vi "PneumaticsMain.vi"(7 "Mode":enum16{"Open", "Control"}(ring)=enum."Control", 8 "error in (no error)":errorcluster, 9 "Value":T1, 10 "Reverse Solenoid Channel":T2=enum."Solenoid 1", 11 "Forward Solenoid Channel":T2) -> (0 "error out":errorcluster)   [LabVIEW 2017]
uses:
  <vilib>/Rock Robotics/WPI/Solenoid/WPI_SolenoidChannel.ctl
  <vilib>/Rock Robotics/WPI/Solenoid/WPI_SolenoidValue.ctl
  <vilib>/Rock Robotics/WPI/Solenoid/WPI_SolenoidOpenDouble.vi
  <vilib>/Rock Robotics/WPI/Solenoid/WPI_SolenoidSetEnum.vi
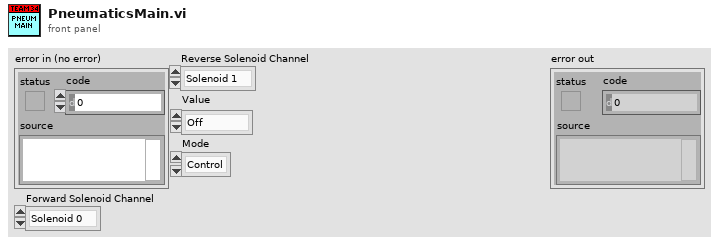
[diagram p1: front panel]
types:
  T1 = typedef "WPI_SolenoidValue.ctl" = enum16{"Off", "On", "Forward", "Reverse"}
  T2 = typedef "WPI_SolenoidChannel.ctl" = enum8{"Solenoid 0", "Solenoid 1", "Solenoid 2", "Solenoid 3", "Solenoid 4", "Solenoid 5", "Solenoid 6", "Solenoid 7", "Invalid"}
  T3 = typedef "WPI_SolenoidDevRef.ctl" = cluster{"DevStatus":errorcluster, "Pneumatics Control Module":u8, "Forward Solenoid Channel":T2, "Reverse Solenoid Channel":T2}
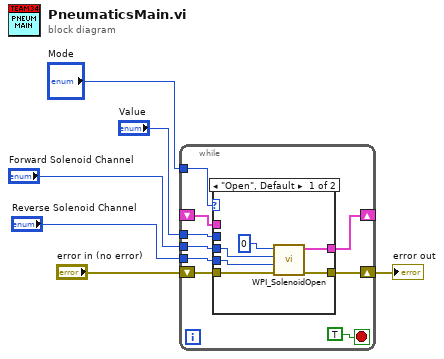
[diagram p0: block diagram]
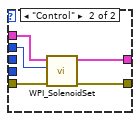
[diagram p2: hidden frame]
diagram:
  n1 = while {
    tunnel: "Mode" -> [w15]
    tunnel: "Forward Solenoid Channel" -> [w13]
    tunnel: "Reverse Solenoid Channel" -> [w12]
    shift-right: [w11] -> _
    shift-left: _ -> [w9]
    tunnel: "Value" -> [w10]
    shift-right: [w14] -> w5
    shift-left: "error in (no error)" -> [w8]
    stop <- TRUE stop-if-true
    n2 = case shown="\"Open\", Default" w15 {
      tunnel: [w20 w23] -> w14
      tunnel: w13 -> [w19 _]
      tunnel: w12 -> [w18 _]
      tunnel: [w17 w24] -> w11
      tunnel: w10 -> [_ w26]
      tunnel: w9 -> [_ w25]
      tunnel: w8 -> [w16 w22]
      frame "Open", Default {
        n3 = call-poly <vilib>:"WPI_SolenoidOpen.vi"("error in (no error)"=w16, "Reverse Solenoid Channel"=w18, "Forward Solenoid Channel"=w19, "Pneumatics Control Module (0)"=u8 0) -> ("error out"=w20:errorcluster, "SolenoidDevRef"=w17:T3)  [unwired: 6 in]
      }
      frame "Control" {
        n4 = call-poly <vilib>:"WPI_SolenoidSet.vi"("error in (no error)"=w22, "Value"=w26, "SolenoidDevRef"=w25) -> ("error out"=w23:errorcluster, "SolenoidDevRef"=w24:T3)  [unwired: 7 in]
      }
    }
  }
  "error out" <- w5
